vi "lj_filter_counter_glitches.vi"(6 "Factor":dbl=2.0 format="%#_13g", 10 "Time":dbl, 11 "Initialized":bool) -> (3 "Valid":bool)   [LabVIEW 2025, in "LabJackEKG.lvlib"]
uses:
  LabJackEKG.lvlib
  <vilib>/ptbypt/NI_PtbyPt.lvlib
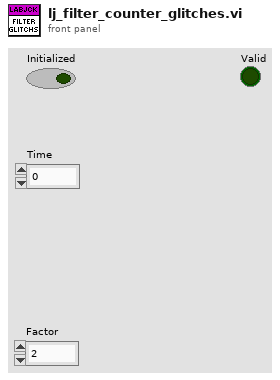
[diagram p1: front panel]
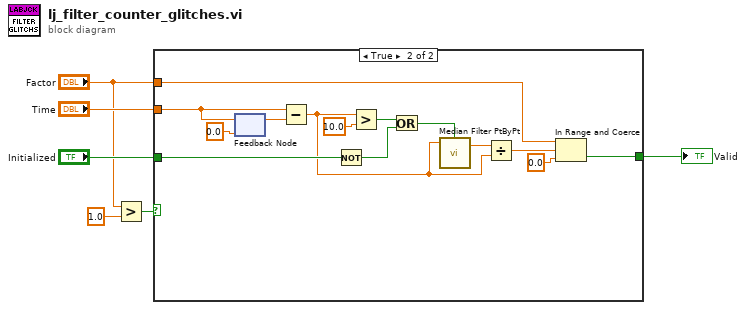
[diagram p0: block diagram]
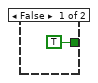
[diagram p2: hidden frame]
diagram:
  n1 = Greater?(x="Factor", y=1.0) -> (0:w2:bool)
  n2 = case shown="True" w2 {
    tunnel: "Initialized" -> [_ w21]
    tunnel: "Time" -> [_ w20]
    tunnel: "Factor" -> [_ w11]
    tunnel: [TRUE w8] -> w4
    frame False {
    }
    frame True {
      n3 = feedback #1(0.0 ("Time")) -> (w19:dbl)
      n4 = feedback-in #1(w20) -> ()
      n5 = Subtract(x=w20, y=w19) -> (x-y=w13:dbl)
      n6 = Not(x=w21) -> (.not. x?=w16:bool)
      n7 = Greater?(x=w13, y=10.0) -> (0:w17:bool)
      n8 = Or(x=w17, y=w16) -> (x .or. y?=w15:bool)
      n9 = call <vilib>:"Median Filter PtByPt.vi"("initialize"=w15, "x"=w13) -> ("Filtered x"=w14:dbl)  [unwired: 2 in, 1 out]
      n10 = Divide(x=w14, y=w13) -> (x/y=w12:dbl)
      n11 = In Range and Coerce(upper limit=w11, x=w12, lower limit=0.0) -> (In Range?=w8:bool)  [unwired: 1 out]
    }
  }
  "Valid" <- w4
